vi "search_command_from_LUT.vi"(2 "parameter_string":string, 3 "input_general_command":string, 4 "input_machine_reference.lvclass":refnum<class "machine.lvclass">) -> (0 "output_specific_command":string, 1 "output_machine_reference.lvclass":refnum<class "machine.lvclass">)   [LabVIEW 2014, in "machine.lvclass"]
uses:
  machine.lvclass
  machine.lvclass/machine.ctl
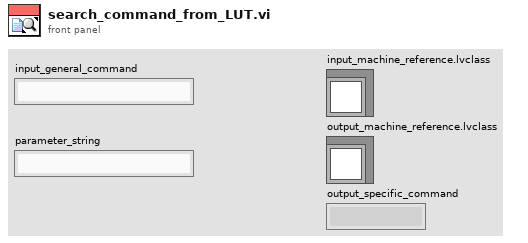
[diagram p1: front panel]
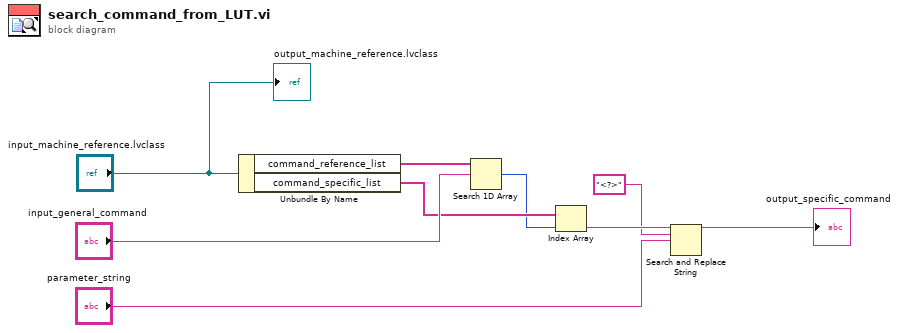
[diagram p0: block diagram]
diagram:
  n1 = Unbundle By Name("input_machine_reference.lvclass") -> ("command_reference_list"=w8:string[], "command_specific_list"=w6:string[])
  n2 = Search 1D Array(1D array=w8, element="input_general_command") -> (index of element=w5:i32)  [unwired: 1 in]
  n3 = Index Array(array=w6, index=w5) -> (element=w4:string)
  n4 = Search and Replace String(input string=w4, search string="<?>", replace string="parameter_string") -> (result string=→"output_specific_command":string)  [unwired: 5 in, 3 out]
  "output_machine_reference.lvclass" <- "input_machine_reference.lvclass"
